vi "Error Process.vi"(8 "error in (no error)":errorcluster, 11 "View Model":T1) -> (0 "error out":errorcluster)   [LabVIEW 2017]
doc: "Centralized error handler of ATM."
uses:
  View Model/Controls/View Model.ctl
  View Model/Controls/Shared Model.ctl
  Controls/Error Model.ctl
  Controls/Error Data.ctl
  Controls/Error Type.ctl
  Controls/Error Source.ctl
  Configuration/Controls/Config Model.ctl
  Configuration/Controls/Config CMD.ctl
  Configuration/Controls/Config Command.ctl
  Controller/Controls/Controller Model.ctl
  Controller/Controls/Controller Overhead.ctl
  Controller/Controls/Controller Transaction.ctl
  Controller/Controls/Controller State.ctl
  Configuration/Controls/Config Data Record.ctl
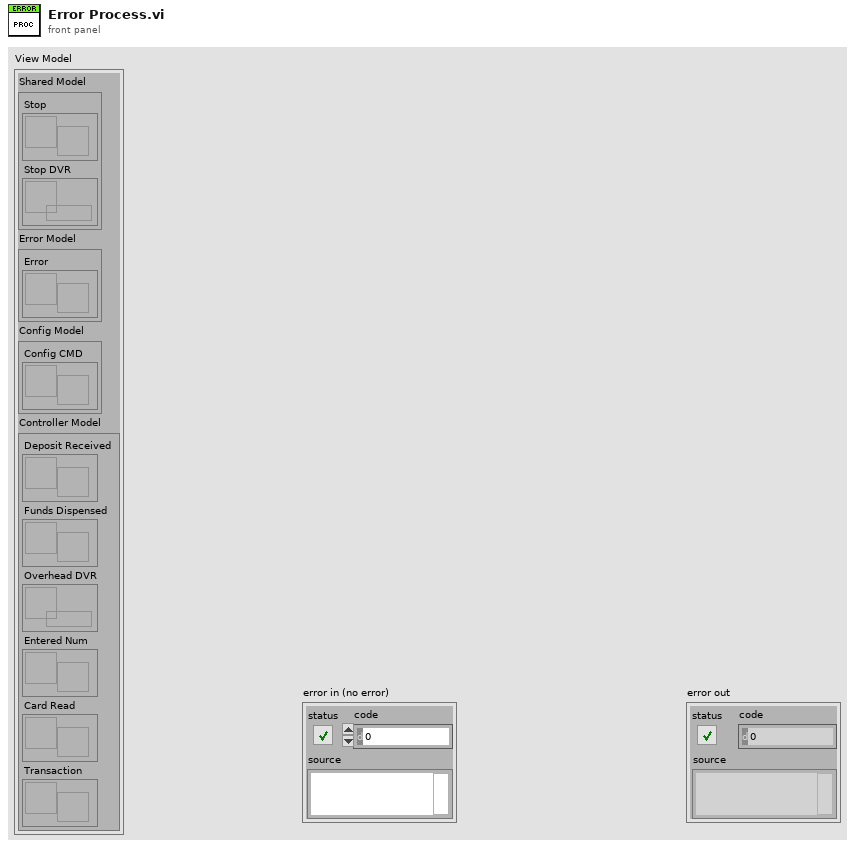
[diagram p1: front panel]
types:
  T1 = typedef "View Model.ctl" = cluster{"Shared Model":T2, "Error Model":T3, "Config Model":T4, "Controller Model":T5}
  T2 = typedef "Shared Model.ctl" = cluster{"Stop":refnum<user-event>, "Stop DVR":refnum<data-value>}
  T3 = typedef "Error Model.ctl" = cluster{"Error":refnum<user-event>}
  T4 = typedef "Config Model.ctl" = cluster{"Config CMD":refnum<user-event>}
  T5 = typedef "Controller Model.ctl" = cluster{"Deposit Received":refnum<user-event>, "Funds Dispensed":refnum<user-event>, "Overhead DVR":refnum<data-value>, "Entered Num":refnum<user-event>, "Card Read":refnum<user-event>, "Transaction":refnum<user-event>}
  T6 = typedef "Error Type.ctl" = enum16{"Console Error", "Sensor Interface IO Error", "Process Step Error"}
  T7 = typedef "Error Source.ctl" = enum16{"User Console", "Display Console", "Sensor Interface"}
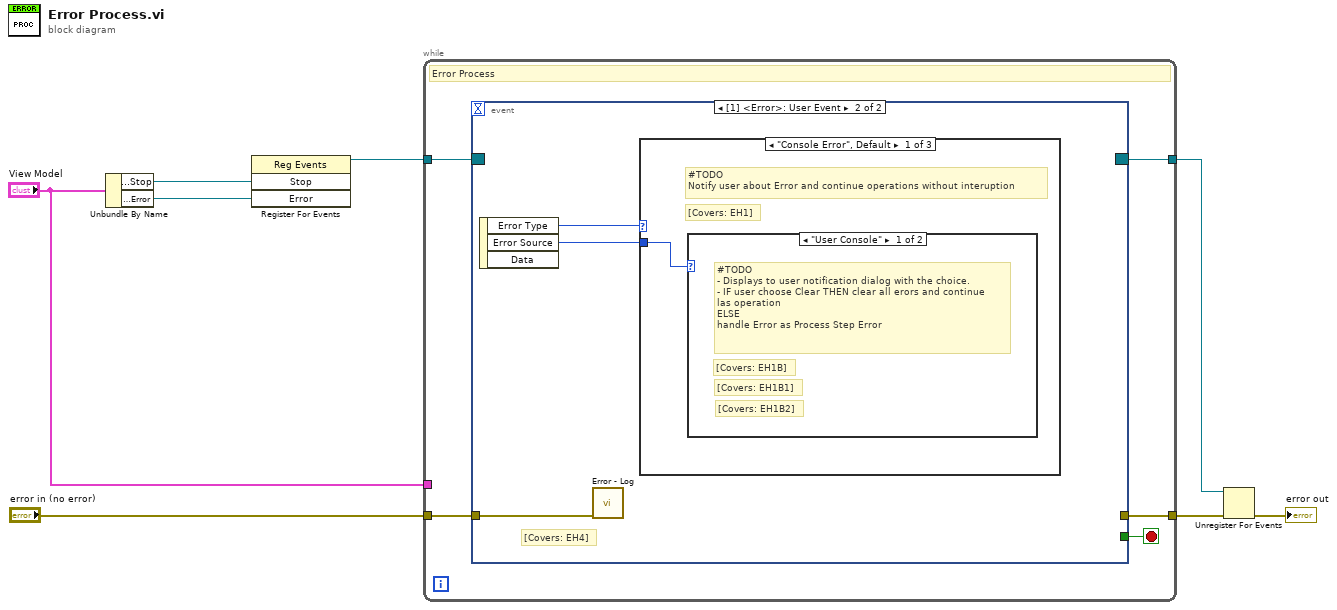
[diagram p0: block diagram]
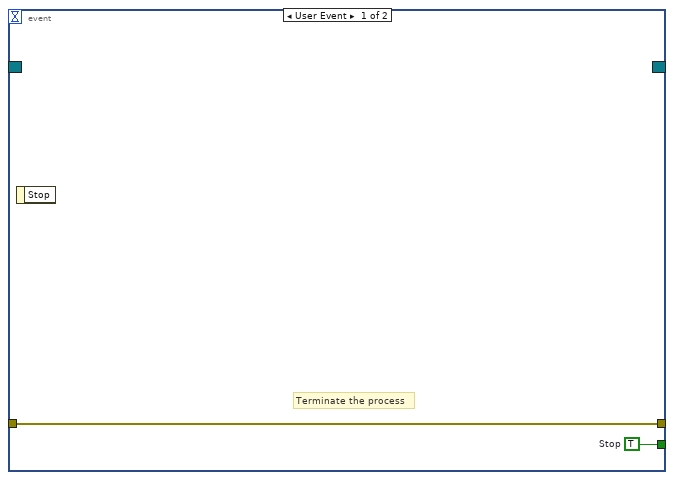
[diagram p2: hidden frame]
diagram:
  n1 = Unbundle By Name("View Model") -> ("Shared Model.Stop"=w8:refnum<user-event>, "Error Model.Error"=w1:refnum<user-event>)
  n2 = register-events(w8, w1) -> (reference out=w7:refnum<event-registration>)  [unwired: 2 in, 1 out]
  n3 = while {
    tunnel: w7 -> [w13]
    tunnel: [w12] -> w6
    tunnel: "error in (no error)" -> [w11]
    tunnel: [w10] -> w3
    tunnel: "View Model" -> [_]
    stop <- w9 stop-if-true
    # "Error Process"
    n4 = event shown="[1] <Error>: User Event" {
      selector: w13 -> [_ _]
      dyn-events: [_ _] -> w12
      timeout: _ -> [_ _]
      tunnel: w11 -> [w15 w16]
      tunnel: [w15 _] -> w10
      tunnel: [w14 _] -> w9
      event User Event {
        w14 = TRUE  # Stop
        # "Terminate the process"
        n5 = event-data() -> ()  [unwired: 1 in, 1 out]
      }
      event User Event {
        # "[Covers: EH4]"
        n6 = event-data() -> ("Error Type"=w17:T6, "Error Source"=w18:T7)  [unwired: 1 in, 1 out]
        n7 = call "Error - Log.vi"("error in (no error)"=w16) -> ()  [unwired: 10 in, 1 out]
        n8 = case shown="\"Console Error\", Default" w17 {
          tunnel: w18 -> [w19 _ _]
          frame "Console Error", Default {
            # "[Covers: EH1]"
            # "#TODO\nNotify user about Error and continue operations without interuption"
            n9 = case shown="\"User Console\"" w19 {
              frame "User Console" {
                # "[Covers: EH1B2]"
                # "[Covers: EH1B1]"
                # "[Covers: EH1B]"
                # "#TODO\n- Displays to user notification dialog with the choice.\n- IF user choose Clear THEN clear all erors and continue\nlas operation\nELSE\nhandle Error as Process Step Error"
              }
              frame "Display Console", Default {
                # "[Covers: EH1A]"
                # "#TODO\nDisplays to user Error dialog. When user click OK\nclears all errors and continues the last operation\nor process step"
              }
            }
          }
          frame "Sensor Interface IO Error" {
            # "[Covers: EH2]"
            # "#TODO\nExecutes Terminate State"
          }
          frame "Process Step Error" {
            # "[Covers: EH3]"
            # "#TODO\nExecutes Terminate State"
          }
        }
      }
    }
  }
  n10 = Unregister For Events(event registration refnum=w6, error in=w3) -> (error out=→"error out":errorcluster)
